vi "校准泵控制.vi"(8 "错误输入（无错误）":errorcluster, 9 "摄氏度":u16, 10 "偏心轮":u16, 11 "枚举":enum16{"进水样", "排液", "加热", "停止"}(ring)) -> (0 "错误输出":errorcluster)   [LabVIEW 2016, in "斯坦道CODMn新电路板.lvlib"]
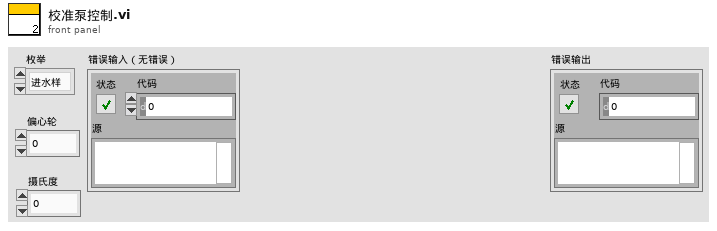
[diagram p1: front panel]
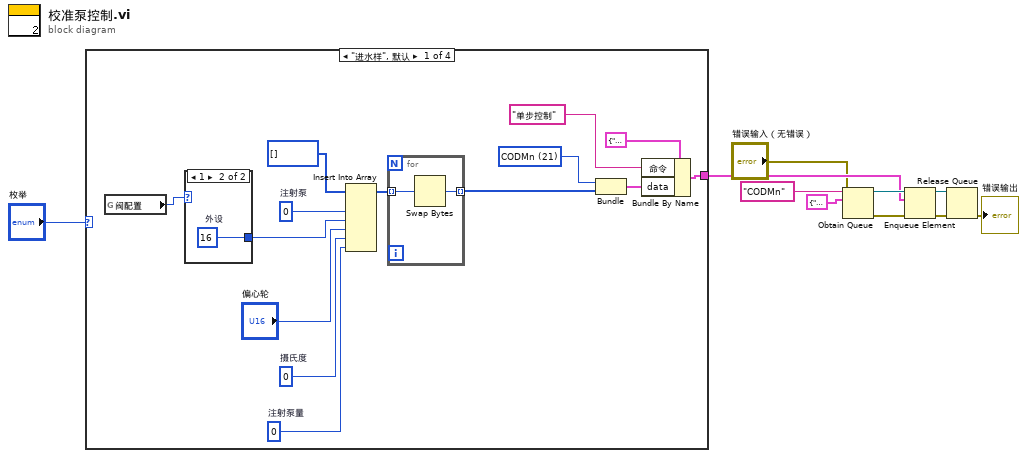
[diagram p0: block diagram]
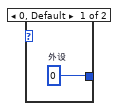
[diagram p2: hidden frame]
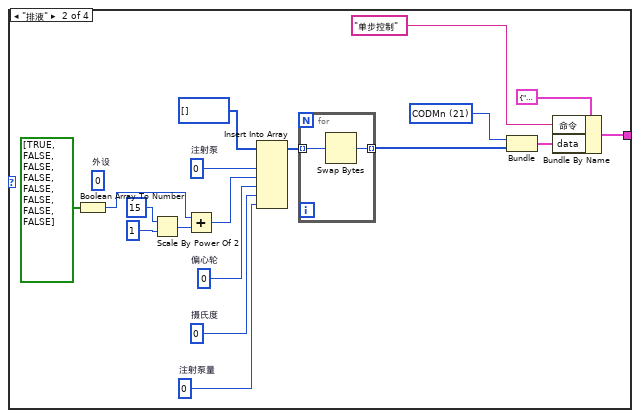
[diagram p3: hidden frame]
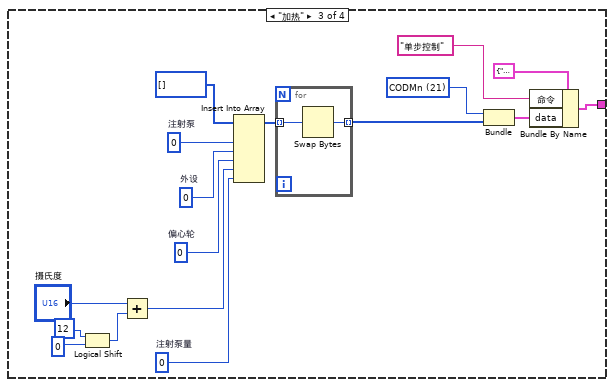
[diagram p4: hidden frame]
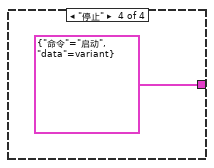
[diagram p5: hidden frame]
diagram:
  n1 = case shown="\"进水样\", 默认" "枚举" {
    tunnel: [w13 w35 w54 cluster{"命令":string, "data":variant} {"命令"="启动", "data"=variant(cluster{"站号":u16, "控制命令":u16[]} {"站号"=21, "控制命令"=[2816]})} ("启动命令")] -> w3
    frame "进水样", Default {
      w18 = u16 21 items=["CODMn"=21, "总磷"=1, "氨氮"=3] ("站号")
      w22 = u16 0  # 注射泵量
      w21 = u16 0  # 摄氏度
      w23 = u16 0  # 注射泵
      n2 = global read "CODMn断电保存全局变量.vi" "阀配置"() -> (w12:u8)
      n3 = case shown="1" w12 {
        tunnel: [w25 w26] -> w11
        frame 0, Default {
          w25 = u16 0  # 外设
        }
        frame 1 {
          w26 = u16 16  # 外设
        }
      }
      n4 = Insert Into Array(array=u16[] [] ("数组"), new element #1=w23, new element #2=w11, new element #3="偏心轮", new element #4=w21, new element #5=w22) -> (w20:u16[])  [unwired: 1 in]
      n5 = for {
        tunnel: w20 -> [w28] mode=indexing
        tunnel: [w27] -> w15 mode=indexing
        n6 = Swap Bytes(anything=w28) -> (byte swapped=w27:u16)
      }
      n7 = Bundle("站号"=w18, w15) -> (w17:cluster{"站号":u16, u16[]})  [unwired: 1 in]
      n8 = Bundle By Name(cluster=cluster{"命令":string, "data":variant} {"命令"="", "data"=variant} ("元素"), "命令"="单步控制", "data"=w17) -> (w13:cluster{"命令":string, "data":variant})
    }
    frame "排液" {
      w40 = u16 21 items=["CODMn"=21, "总磷"=1, "氨氮"=3] ("站号")
      w44 = u16 0  # 注射泵量
      w43 = u16 0  # 摄氏度
      w41 = u16 0  # 偏心轮
      (unwired) u16 0  # 外设
      w45 = u16 0  # 注射泵
      n9 = Boolean Array To Number ("布尔数组至数值转换")(Boolean array=bool[] [TRUE, FALSE, FALSE, FALSE, FALSE, FALSE, FALSE, FALSE] ("添加的数组")) -> (number=w34:u16)
      n10 = Scale By Power Of 2(n=i16 15, x=u16 1 ("y")) -> (x*2^n=w33:u16)
      n11 = Add(x=w34, y=w33) -> (x+y=w29:u16)
      n12 = Insert Into Array(array=u16[] [] ("数组"), new element #1=w45, new element #2=w29, new element #3=w41, new element #4=w43, new element #5=w44) -> (w42:u16[])  [unwired: 1 in]
      n13 = for {
        tunnel: w42 -> [w48] mode=indexing
        tunnel: [w47] -> w37 mode=indexing
        n14 = Swap Bytes(anything=w48) -> (byte swapped=w47:u16)
      }
      n15 = Bundle("站号"=w40, w37) -> (w39:cluster{"站号":u16, u16[]})  [unwired: 1 in]
      n16 = Bundle By Name(cluster=cluster{"命令":string, "data":variant} {"命令"="", "data"=variant} ("元素"), "命令"="单步控制", "data"=w39) -> (w35:cluster{"命令":string, "data":variant})
    }
    frame "加热" {
      w59 = u16 21 items=["CODMn"=21, "总磷"=1, "氨氮"=3] ("站号")
      w62 = u16 0  # 注射泵量
      w60 = u16 0  # 偏心轮
      w63 = u16 0  # 外设
      w64 = u16 0  # 注射泵
      n17 = Logical Shift(y=i16 12, x=i16 0) -> (x << y=w52:i16)
      n18 = Add(x="摄氏度", y=w52) -> (x+y=w49:u16)
      n19 = Insert Into Array(array=u16[] [] ("数组"), new element #1=w64, new element #2=w63, new element #3=w60, new element #4=w49, new element #5=w62) -> (w61:u16[])  [unwired: 1 in]
      n20 = for {
        tunnel: w61 -> [w67] mode=indexing
        tunnel: [w66] -> w56 mode=indexing
        n21 = Swap Bytes(anything=w67) -> (byte swapped=w66:u16)
      }
      n22 = Bundle("站号"=w59, w56) -> (w58:cluster{"站号":u16, u16[]})  [unwired: 1 in]
      n23 = Bundle By Name(cluster=cluster{"命令":string, "data":variant} {"命令"="", "data"=variant} ("元素"), "命令"="单步控制", "data"=w58) -> (w54:cluster{"命令":string, "data":variant})
    }
    frame "停止" {
    }
  }
  n24 = Obtain Queue(name (unnamed)="CODMn" ("名称（未命名）"), element data type=cluster{"命令":string, "data":variant} {"命令"="", "data"=variant}, error in (no error)="错误输入（无错误）") -> (queue out=w8:refnum<queue>, error out=w7:errorcluster)  [unwired: 2 in, 1 out]
  n25 = Enqueue Element(queue=w8, element=w3, error in (no error)=w7) -> (queue out=w6:refnum<queue>, error out=w5:errorcluster)  [unwired: 1 in, 1 out]
  n26 = Release Queue(queue=w6, error in (no error)=w5) -> (error out=→"错误输出":errorcluster)  [unwired: 1 in, 2 out]
